vi "总磷数据时间处理.vi"(9 "已对齐时间输入":T1 {"单位" items=["ug/L", "mg/L", "ppm", "mg/m3", "cm", "ppb", "ug/m3", "%", "nmol/mol", "umol/mol", "MPN/L", "MPN/100ml", "ng/m3", "NTU", "无量纲", "ms/cm", "us/cm", "℃", "mV", "万个/L"]}, 10 "对齐参考时间":T1 {"单位" items=["ug/L", "mg/L", "ppm", "mg/m3", "cm", "ppb", "ug/m3", "%", "nmol/mol", "umol/mol", "MPN/L", "MPN/100ml", "ng/m3", "NTU", "无量纲", "ms/cm", "us/cm", "℃", "mV", "万个/L"]}, 11 "待对齐时间":T1 {"单位" items=["ug/L", "mg/L", "ppm", "mg/m3", "cm", "ppb", "ug/m3", "%", "nmol/mol", "umol/mol", "MPN/L", "MPN/100ml", "ng/m3", "NTU", "无量纲", "ms/cm", "us/cm", "℃", "mV", "万个/L"]}) -> (3 "已对齐时间输出":T1 {"单位" items=["ug/L", "mg/L", "ppm", "mg/m3", "cm", "ppb", "ug/m3", "%", "nmol/mol", "umol/mol", "MPN/L", "MPN/100ml", "ng/m3", "NTU", "无量纲", "ms/cm", "us/cm", "℃", "mV", "万个/L"]})   [LabVIEW 2016, in "斯坦道总磷.lvlib"]
panel:
  out "数字":u32
  out "数组":timestamp[](array[timestamp])
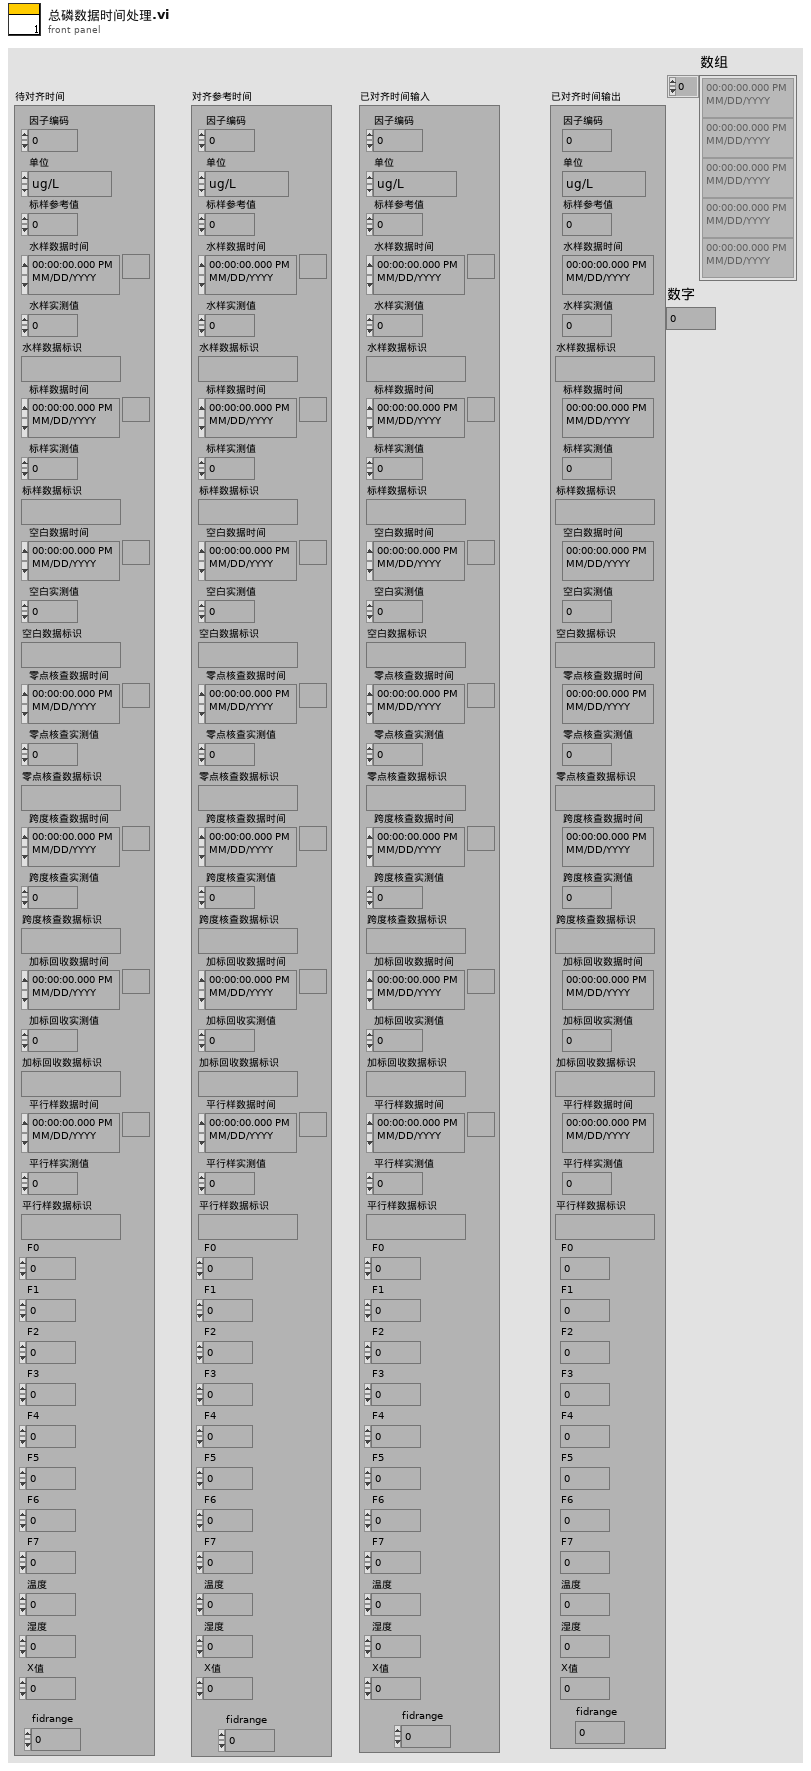
[diagram p1: front panel]
types:
  T1 = cluster{"因子编码":u32, "单位":u16, "标样参考值":sgl, "水样数据时间":timestamp, "水样实测值":sgl, "水样数据标识":string, "标样数据时间":timestamp, "标样实测值":sgl, "标样数据标识":string, "空白数据时间":timestamp, "空白实测值":sgl, "空白数据标识":string, "零点核查数据时间":timestamp, "零点核查实测值":sgl, "零点核查数据标识":string, "跨度核查数据时间":timestamp, "跨度核查实测值":sgl, "跨度核查数据标识":string, "加标回收数据时间":timestamp, "加标回收实测值":sgl, "加标回收数据标识":string, "平行样数据时间":timestamp, "平行样实测值":sgl, "平行样数据标识":string, "F0":sgl, "F1":sgl, "F2":sgl, "F3":sgl, "F4":sgl, "F5":sgl, "F6":sgl, "F7":sgl, "温度":sgl, "湿度":sgl, "X值":sgl, "fidrange":u16}
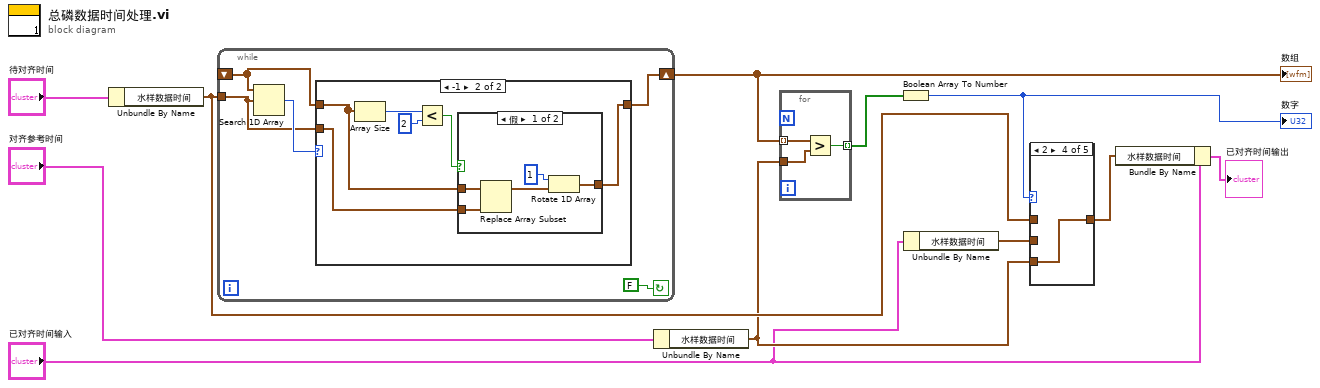
[diagram p0: block diagram]
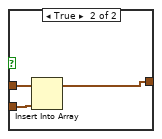
[diagram p7: hidden frame]
diagram:
  n1 = Unbundle By Name("待对齐时间") -> ("水样数据时间"=w7:timestamp)
  n2 = while {
    shift-right: [w13] -> w9
    shift-left: _ -> [w15]
    tunnel: w7 -> [w14]
    stop <- FALSE continue-if-true
    n3 = Search 1D Array(1D array=w15, element=w14) -> (index of element=w16:i32)  [unwired: 1 in]
    n4 = case shown="-1" w16 {
      tunnel: w15 -> [w17 w21]
      tunnel: w14 -> [_ w23]
      tunnel: [w17 w22] -> w13
      frame 0, Default {
      }
      frame -1 {
        n5 = Array Size(array=w21) -> (size(s)=w20:i32)
        n6 = Less?(x=w20, y=2) -> (x < y?=w18:bool)
        n7 = case shown="假" w18 {
          tunnel: w23 -> [w28 w31]
          tunnel: [w24 w30] -> w22
          tunnel: w21 -> [w26 w29]
          frame False {
            n8 = Replace Array Subset(array=w26, new element=w28) -> (w25:timestamp[])  [unwired: 1 in]
            n9 = Rotate 1D Array(1:w25, 2:1 ("n")) -> (0:w24:timestamp[])
          }
          frame True {
            n10 = Insert Into Array(array=w29, new element=w31) -> (w30:timestamp[])  [unwired: 1 in]
          }
        }
      }
    }
  }
  "数组" <- w9
  n11 = Unbundle By Name("对齐参考时间") -> ("水样数据时间"=w6:timestamp)
  n12 = for {
    tunnel: w9 -> [w34] mode=indexing
    tunnel: w6 -> [w33]
    tunnel: [w32] -> w8 mode=indexing
    n13 = Greater?(x=w34, y=w33) -> (0:w32:bool)
  }
  n14 = Boolean Array To Number(Boolean array=w8) -> (number=w5:u32)
  "数字" <- w5
  n15 = Unbundle By Name("已对齐时间输入") -> ("水样数据时间"=w4:timestamp)
  n16 = case shown="2" w5 {
    tunnel: [w35 w36 w37 w38 w39] -> w2
    tunnel: w7 -> [w35 _ _ _ w39]
    tunnel: w6 -> [_ _ w37 w38 _]
    tunnel: w4 -> [_ w36 _ _ _]
    frame Default {
    }
    frame 0 {
    }
    frame 1 {
    }
    frame 2 {
    }
    frame 3 {
    }
  }
  n17 = Bundle By Name(cluster="已对齐时间输入", "水样数据时间"=w2) -> (→"已对齐时间输出":T1)
